vi "FGV-MassData(lvlibp).vi"(6 "Operation":T1, 8 "Error in":errorcluster caption="Error in (no error)", 9 "size":i32, 10 "Start":i32, 11 "Data in":u8[](array[numeric])) -> (0 "Error out":errorcluster, 1 "Active Read Oper":T2, 2 "Active Write Oper":T2, 3 "Data out":u8[](array[numeric]))   [LabVIEW 2017, in "CSM MassData Parameter Support.lvlib"]
uses:
  CSM MassData Parameter Support.lvlib
  Def-MassDataOper-Status.ctl
  Operation-FGV-MassData.ctl
  FGV-MassData.vi
  <userlib>/_NEVSTOP/Communicable State Machine(CSM)/Communicable State Machine.lvlib
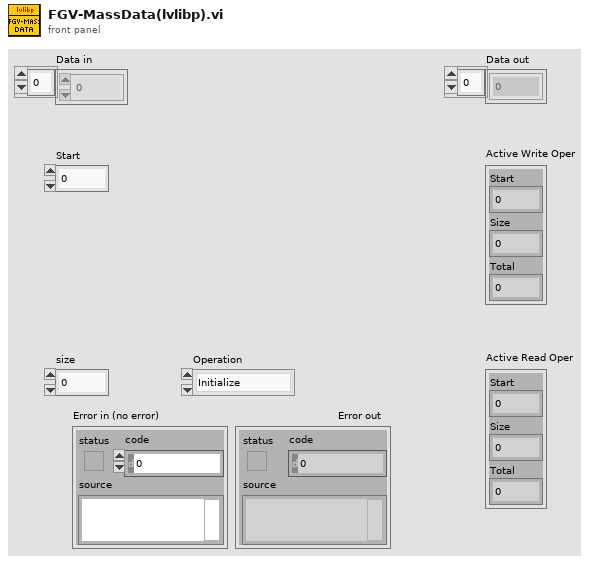
[diagram p1: front panel]
types:
  T1 = typedef "CSM MassData Parameter Support.lvlib/Operation-FGV-MassData.ctl" = enum16{"Initialize", "Read", "Write", "Status", "Release"}
  T2 = typedef "CSM MassData Parameter Support.lvlib/Def-MassDataOper-Status.ctl" = cluster{"Start":i32, "Size":i32, "Total":i32}
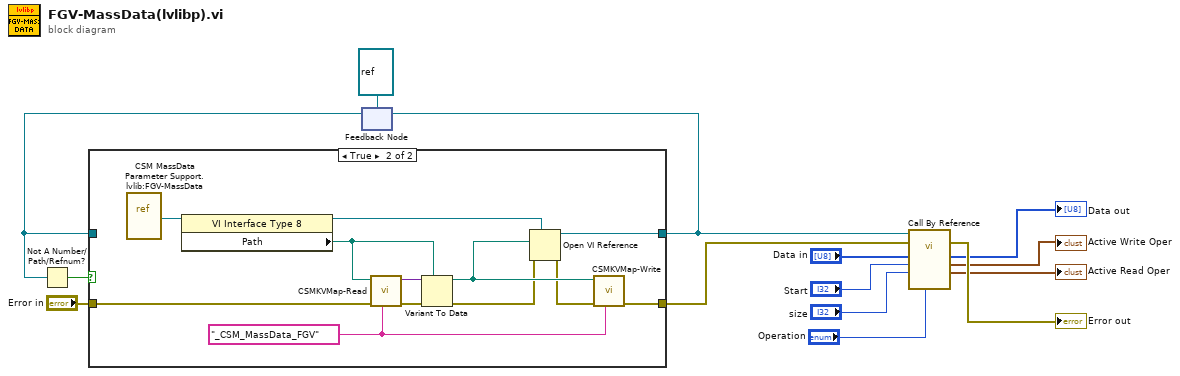
[diagram p0: block diagram]
diagram:
  n1 = feedback #1(refnum<vi> refnum) -> (w12:refnum<vi>)
  n2 = Not A Number/Path/Refnum?(number/path/refnum=w12) -> (NaN/Path/Refnum?=w13:bool)
  n3 = case shown="True" w13 {
    tunnel: [w16 w20] -> w11
    tunnel: w12 -> [w16 _]
    tunnel: "Error in" -> [w15 w19]
    tunnel: [w15 w18] -> w9
    frame False {
    }
    frame True {
      w17 = "_CSM_MassData_FGV" ("name")
      n4 = vi-ref "CSM MassData Parameter Support.lvlib:FGV-MassData.vi"() -> (w28:refnum<vi>)
      n5 = property class="VI Interface Type 8"(reference=w28) -> (reference out=w21:refnum<vi>, "Path"=w25:path)  [unwired: 1 in, 1 out]
      n6 = call <userlib>:"CSMKVMap-Read.vi"("name"=w17, "Error in"=w19, "default value (empty variant)"=w25) -> ("Error out"=w27:errorcluster, "value"=w26:variant)  [unwired: 5 in]
      n7 = Variant To Data(error in=w27, type=w25, Variant=w26) -> (data=w24:path, error out=w22:errorcluster)
      n8 = Open VI Reference(type specifier VI Refnum (for type only)=w21, vi path=w24, error in (no error)=w22) -> (vi reference=w20:refnum<vi>, error out=w23:errorcluster)  [unwired: 3 in]
      n9 = call <userlib>:"CSMKVMap-Write.vi"("name"=w17, "Error in"=w23, "value"=w24) -> ("Error out"=w18:errorcluster)  [unwired: 6 in]
    }
  }
  n10 = feedback-in #1(w11) -> ()
  n11 = call-by-ref "?"(reference=w11, error in=w9, "Operation"="Operation", "size"="size", "Start"="Start", "Data in"="Data in") -> (error out=→"Error out":errorcluster, "Active Read Oper"=→"Active Read Oper":T2, "Active Write Oper"=→"Active Write Oper":T2, "Data out"=→"Data out":u8[])  [unwired: 4 in, 2 out]
